vi "DeleteAndAdd.vi"(0 "Input":dbl[][](array[numeric])=[[nan, 1.0, nan, nan, nan, 5.0, 6.0, nan, nan, nan, 10.0], [nan, nan, nan, nan, nan, nan, nan, nan, nan, nan, nan], [nan, nan, nan, nan, nan, nan, nan, nan, nan, nan, nan], [nan, nan, nan, nan, nan, nan, nan, nan, nan, nan, nan], [nan, nan, nan, nan, nan, nan, nan, nan, nan, nan, nan], [nan, nan, nan, nan, nan, nan, nan, nan, nan, nan, nan], [nan, nan, nan, nan, nan, nan, nan, nan, nan, nan, nan], [nan, nan, nan, nan, nan, nan, nan, nan, nan, nan, nan], [nan, nan, nan, nan, nan, nan, nan, nan, nan, nan, nan], [nan, nan, nan, nan, nan, nan, nan, nan, nan, nan, nan]], 1 "Old Initialization Data":T2, 2 "New Initialization Data":T2, 3 "ColumnSize":i32, 4 "RowSize":i32, 5 "error in (no error)":errorcluster, 7 "StatDataIn":T1(array[cluster])) -> (13 "StatDataOut":T1(array[cluster]), 14 "Output 2 After Adding":dbl[][](array[numeric]), 19 "error out":errorcluster)   [LabVIEW 2019, in "Zen Analytics.lvlib" / "Zen Analytics.lvclass"]
uses:
  Zen Analytics.lvclass
panel:
  out "Disabled Meaurement ID":i32[](array[numeric])
  out "Array":bool[](array[boolean])
  out "Add Column":i32[](array[numeric])
  out "Delete Column":i32[](array[numeric])
  out "Output 1 - After Delete":dbl[][](array[numeric])
types:
  T1 = cluster{"SumOfSquareOfData":dbl, "SumOfMeasurementData":dbl, "N ":u32}[]
  T2 = cluster{"Measurement-ID":i32[], "Measurement Names":string[], "NominalValues":dbl[], "LSL":dbl[], "USL":dbl[], "LCL":dbl[], "UCL":dbl[]}
  T3 = cluster{"SumOfSquareOfData":dbl, "SumOfMeasurementData":dbl, "N ":u32}
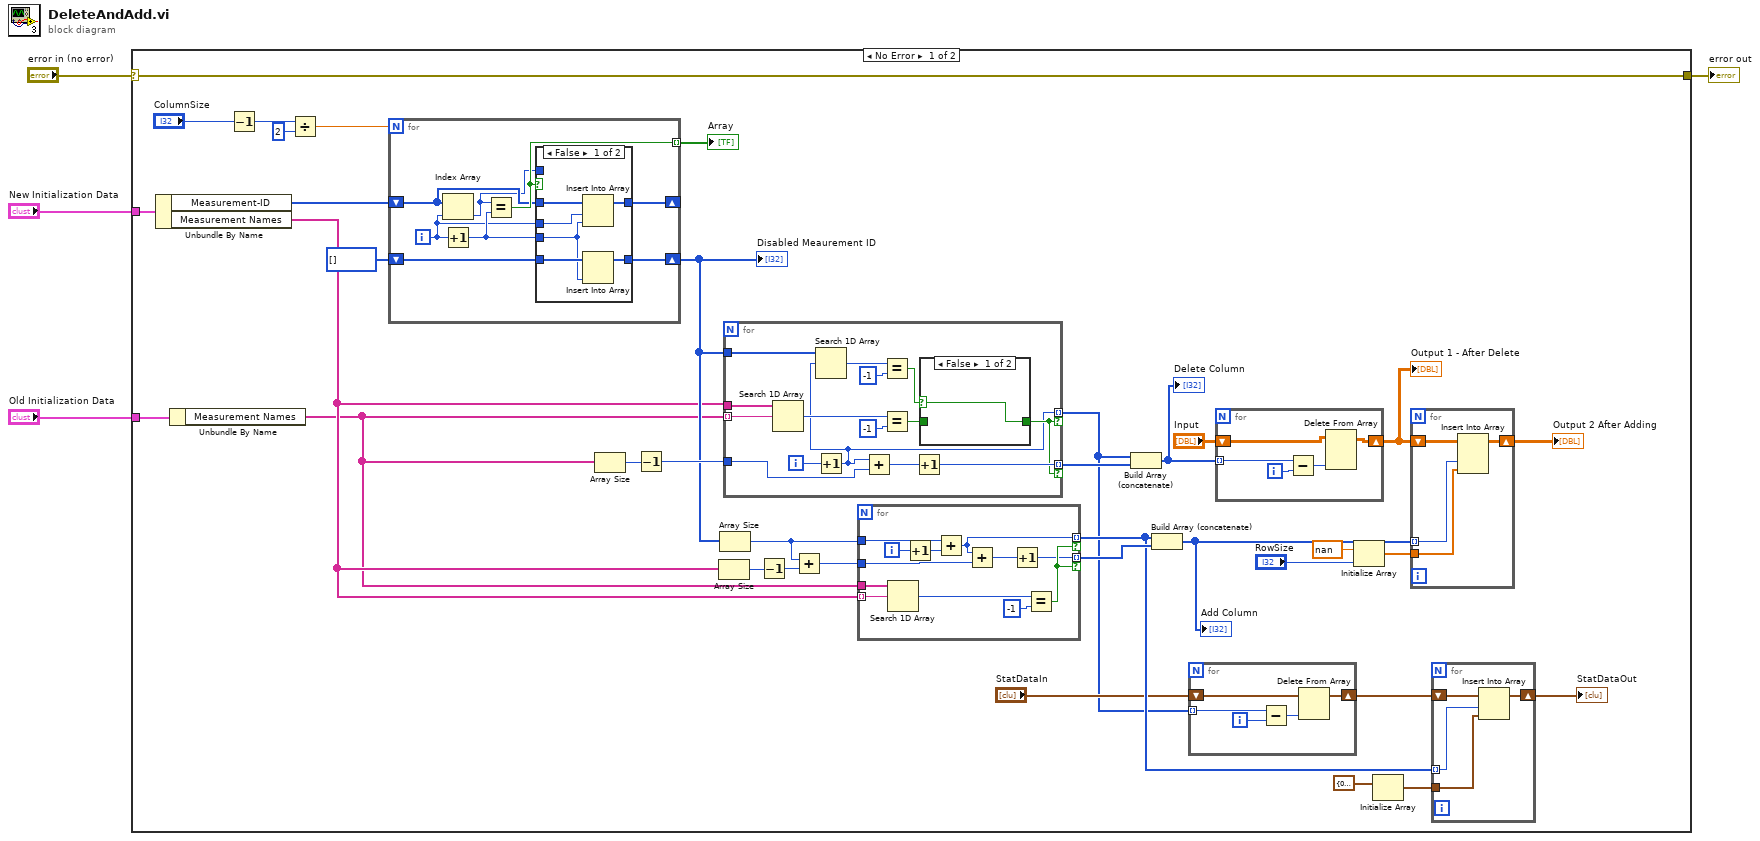
[diagram p0: block diagram]
diagram:
  n1 = case shown="No Error" "error in (no error)" {
    selector: "error in (no error)" -> [w37 w104]
    tunnel: [w37 w104] -> w3
    tunnel: "New Initialization Data" -> [w16 _]
    tunnel: "Old Initialization Data" -> [w13 _]
    frame No Error {
      n2 = Unbundle By Name(w16) -> ("Measurement-ID"=w15:i32[], "Measurement Names"=w14:string[])
      n3 = Unbundle By Name(w13) -> ("Measurement Names"=w12:string[])
      n4 = Decrement(x="ColumnSize") -> (x-1=w27:i32)
      n5 = Divide(x=w27, y=2) -> (x/y=w25:dbl)
      n6 = for {
        N: w25 -> [_]
        tunnel: [w57] -> w24 mode=indexing
        shift-right: [w55] -> w20
        shift-left: i32[] [] ("New Meaurement ID") -> [w56]
        shift-right: [w50] -> _
        shift-left: w15 -> [w53]
        i -> [w51]
        n7 = Index Array(array=w53, index=w51) -> (element=w52:i32)
        n8 = Increment(x=w51) -> (x+1=w54:i32)
        n9 = Equal?(x=w52, y=w54) -> (x = y?=w57:bool)
        n10 = case shown="False" w57 {
          tunnel: w56 -> [w63 w65]
          tunnel: [w62 w65] -> w55
          tunnel: w54 -> [w58 _]
          tunnel: w53 -> [w61 w64]
          tunnel: w52 -> [_ _]
          tunnel: w51 -> [w60 _]
          tunnel: [w59 w64] -> w50
          frame False {
            n11 = Insert Into Array(array=w61, index=w60, new element=w58) -> (w59:i32[])
            n12 = Insert Into Array(array=w63, new element=w58) -> (w62:i32[])  [unwired: 1 in]
          }
          frame True {
          }
        }
      }
      "Array" <- w24
      "Disabled Meaurement ID" <- w20
      n13 = Array Size(array=w12) -> (size(s)=w40:i32)
      n14 = Decrement(x=w40) -> (x-1=w39:i32)
      n15 = Array Size(array=w14) -> (size(s)=w36:i32)
      n16 = Array Size(array=w20) -> (size(s)=w19:i32)
      n17 = for {
        tunnel: w14 -> [w100]
        tunnel: w12 -> [w99] mode=indexing
        tunnel: [w87] -> w5 mode=indexing if=w88
        tunnel: w39 -> [w97]
        tunnel: [w95] -> w38 mode=indexing if=w88
        tunnel: w20 -> [w94]
        i -> [w93]
        n18 = Search 1D Array(1D array=w100, element=w99) -> (index of element=w101:i32)  [unwired: 1 in]
        n19 = Increment(x=w93) -> (x+1=w87:i32)
        n20 = Search 1D Array(1D array=w94, element=w87) -> (index of element=w92:i32)  [unwired: 1 in]
        n21 = Add(x=w87, y=w97) -> (x+y=w96:i32)
        n22 = Equal?(x=w92, y=-1) -> (x = y?=w90:bool)
        n23 = Equal?(x=w101, y=-1) -> (x = y?=w89:bool)
        n24 = Increment(x=w96) -> (x+1=w95:i32)
        n25 = case shown="False" w90 {
          selector: w90 -> [w102 _]
          tunnel: [w102 w103] -> w88
          tunnel: w89 -> [_ w103]
          frame False {
          }
          frame True {
          }
        }
      }
      n26 = Decrement(x=w36) -> (x-1=w18:i32)
      n27 = Add(x=w19, y=w18) -> (x+y=w17:i32)
      n28 = for {
        tunnel: w12 -> [w80]
        tunnel: w14 -> [w79] mode=indexing
        tunnel: [w70] -> w8 mode=indexing if=w75
        tunnel: w17 -> [w77]
        tunnel: [w74] -> w35 mode=indexing if=w75
        tunnel: w19 -> [w72]
        i -> [w73]
        n29 = Search 1D Array(1D array=w80, element=w79) -> (index of element=w81:i32)  [unwired: 1 in]
        n30 = Increment(x=w73) -> (x+1=w71:i32)
        n31 = Add(x=w72, y=w71) -> (x+y=w70:i32)
        n32 = Add(x=w70, y=w77) -> (x+y=w76:i32)
        n33 = Increment(x=w76) -> (x+1=w74:i32)
        n34 = Equal?(x=w81, y=-1) -> (x = y?=w75:bool)
      }
      n35 = Build Array (concatenate)(w5, w38) -> (w22:i32[])
      "Delete Column" <- w22
      n36 = Build Array (concatenate)(w8, w35) -> (w21:i32[])
      "Add Column" <- w21
      n37 = for {
        tunnel: w5 -> [w42] mode=indexing
        shift-right: [w44] -> w6
        shift-left: "StatDataIn" -> [w45]
        i -> [w43]
        n38 = Subtract(x=w42, y=w43) -> (x-y=w41:i32)
        n39 = Delete From Array(array=w45, index=w41) -> (array with subset deleted=w44:T1)  [unwired: 1 in, 1 out]
      }
      n40 = for {
        tunnel: w22 -> [w83] mode=indexing
        shift-right: [w85] -> w31
        shift-left: "Input" -> [w86]
        i -> [w84]
        n41 = Subtract(x=w83, y=w84) -> (x-y=w82:i32)
        n42 = Delete From Array(array=w86, index (col)=w82) -> (array with subset deleted=w85:dbl[][])  [unwired: 2 in, 1 out]
      }
      "Output 1 - After Delete" <- w31
      n43 = Initialize Array(nan ("element"), "RowSize") -> (w33:dbl[])
      n44 = Initialize Array(T3 {"SumOfSquareOfData"=0.0, "SumOfMeasurementData"=0.0, "N "=0} ("Cluster")) -> (w9:T1)  [unwired: 1 in]
      n45 = for {
        tunnel: w33 -> [w69]
        shift-right: [w68] -> w30
        shift-left: w31 -> [w67]
        tunnel: w21 -> [w66] mode=indexing
        n46 = Insert Into Array(array=w67, index (col)=w66, new element=w69) -> (w68:dbl[][])  [unwired: 1 in]
      }
      "Output 2 After Adding" <- w30
      n47 = for {
        tunnel: w9 -> [w46]
        shift-right: [w49] -> w11
        shift-left: w6 -> [w48]
        tunnel: w8 -> [w47] mode=indexing
        n48 = Insert Into Array(array=w48, index=w47, new element=w46) -> (w49:T1)
      }
      "StatDataOut" <- w11
    }
    frame Error {
    }
  }
  "error out" <- w3
